vi "GL_response.vi"() -> ()   [LabVIEW 2020]
panel:
  out "Response":string
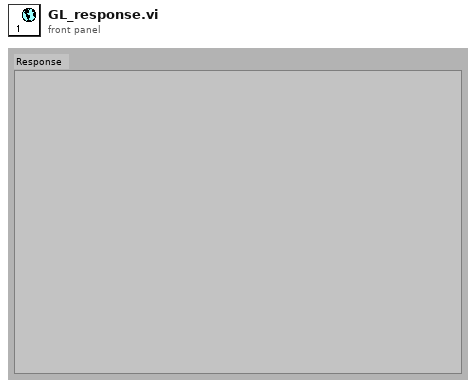
[diagram p1: front panel]
diagram:
